vi "ExSubSetupSimple.vi"(2 "error in (no error)":errorcluster, 3 "Close comp time":u32, 4 "Open comp time":u32=8, 5 "Camera Handle":u32) -> (0 "error out":errorcluster, 1 "Camera Handle":u32)   [LabVIEW 2010]
panel:
  # "ExSubSetupSimple:\nThis Sub VI sets up the skips, cleans, and shutter parameters.\nThis should be changed to suit the camera you are using."
  # "Note: for Cascade and PhotonMax these\nshould be zero."
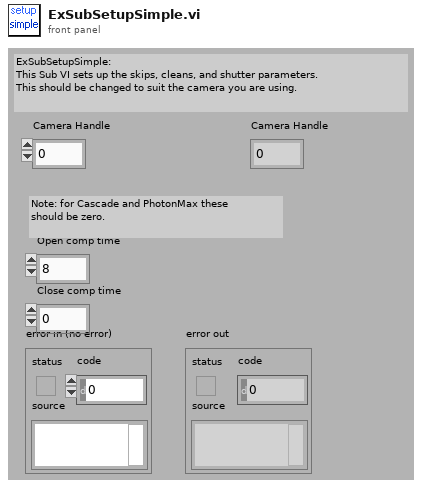
[diagram p1: front panel]
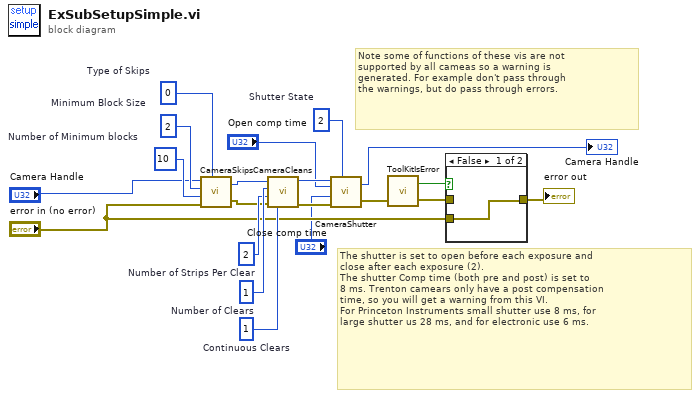
[diagram p0: block diagram]
diagram:
  w12 = u32 0  # Type of Skips
  w13 = u32 2  # Minimum Block Size
  w11 = u32 10  # Number of Minimum blocks
  w15 = u32 1  # Number of Clears
  w14 = u32 2  # Number of Strips Per Clear
  w16 = u32 1  # Continuous Clears
  w17 = u32 2  # Shutter State
  # "Note some of functions of these vis are not \nsupported by all cameas so a warning is \ngenerated. For example don't pass through \nthe warnings, but do pass through errors."
  # "The shutter is set to open before each exposure and\nclose after each exposure (2).\nThe shutter Comp time (both pre and post) is set to \n8 ms. Trenton camears only have a post compensation \ntime, so you will get a warning from this VI.\nFor Princeton Instruments small shutter use 8 ms, for \nlarge shutter us 28 ms, and for electronic use 6 ms."
  n1 = call <userlib>:"CameraSkips.vi"("Camera Handle"="Camera Handle", "Minimum Block Size"=w13, "Number of Minimum blocks"=w11, "error in"="error in (no error)", "Type of Skips"=w12) -> ("Camera Handle"=w10:u32, "error out"=w9:errorcluster)
  n2 = call <userlib>:"CameraCleans.vi"("Camera Handle"=w10, "Number of Clears"=w15, "Number of Strips Per Clear"=w14, "error in"=w9, "Continuous Clears"=w16) -> ("Camera Handle"=w18:u32, "error out"=w19:errorcluster)
  n3 = call <userlib>:"CameraShutter.vi"("Camera Handle"=w18, "Shutter Comp Time: Pre Open"="Open comp time", "Shutter Comp Time: Post Open"="Close comp time", "error in"=w19, "Shutter State"=w17) -> ("Camera Handle"=→"Camera Handle":u32, "error out"=w7:errorcluster)
  n4 = call <userlib>:"ToolKitIsError.vi"("error in"=w7) -> ("error out"=w5:errorcluster, "Error Flag"=w6:bool)  [unwired: 1 in]
  n5 = case shown="False" w6 {
    tunnel: w5 -> [_ w22]
    tunnel: [w21 w22] -> w4
    tunnel: "error in (no error)" -> [w21 _]
    frame False {
    }
    frame True {
    }
  }
  "error out" <- w4
